vi "Configure Data Storage.vi"(5 "Trigger Scan Mode (F: Off)":bool, 7 "Acquisition Mode (T: One-Shot)":bool=TRUE, 8 "Error In (no error)":errorcluster, 10 "Data Sample Rate (0: 62.5 mHz)":u16(ring) items=["62.5 mHz", "125 mHz", "250 mHz", "500 mHz", "1 Hz", "2 Hz", "4 Hz", "8 Hz", "16 Hz", "32 Hz", "64 Hz", "128 Hz", "256 Hz", "512 Hz", "Trigger"], 11 "VISA Resource Name":refnum<visa-resource-name>) -> (0 "Error Out":errorcluster, 3 "VISA Resource Name Out":refnum<visa-resource-name>)   [LabVIEW 2010, in "Stanford Research 844.lvlib"]
doc: "This VI configures data storage."
uses:
  <instrlib>/Stanford Research 844/Stanford Research 844.lvlib
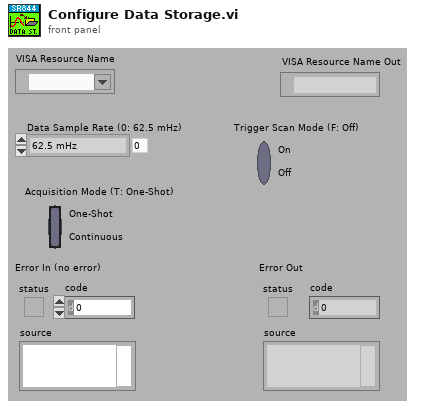
[diagram p1: front panel]
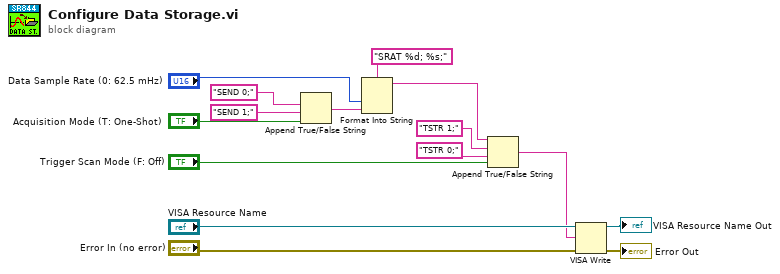
[diagram p0: block diagram]
diagram:
  n1 = Append True/False String(1:"Acquisition Mode (T: One-Shot)", 2:"SEND 1;" ("true string"), 3:"SEND 0;" ("true string")) -> (0:w4:string)  [unwired: 1 in]
  n2 = Format Into String(format string="SRAT %d; %s;", "Data Sample Rate (0: 62.5 mHz)", w4) -> (resulting string=w8:string)  [unwired: 2 in, 1 out]
  n3 = Append True/False String(1:"Trigger Scan Mode (F: Off)", 2:"TSTR 0;" ("true string"), 3:"TSTR 1;" ("true string"), 4:w8) -> (0:w1:string)
  n4 = VISA Write(VISA resource name="VISA Resource Name", write buffer=w1, error in (no error)="Error In (no error)") -> (VISA resource name out=→"VISA Resource Name Out":refnum<visa-resource-name>, error out=→"Error Out":errorcluster)  [unwired: 1 out]
